vi "Build Result Array from Shots.vi"(7 "Stages":T1[](array[typedef]), 8 "Injection Event Dwell Period (ms)":dbl, 10 "Injection Event Count":u32, 11 "Shot Info Array":T5[](array[typedef]) {"Results"."Off-Stage Min Volt" format="%#.6g"; "Results"."Off-Stage Avg Volt" format="%#.6g"; "Results"."Off-Stage Max Volt" format="%#.6g"; "Results"."Total Stage Time (us)" format="%#.6g"; "Results"."Off-Stage Avg Current" format="%#.6g"; "Results"."Total Voltage Pulses" format="%#.6g"; "Results"."Off-Stage Min Current" format="%#.6g"; "Results"."Off-Stage Max Current" format="%#.6g"}) -> (1 "Result Array":dbl[](array[numeric]))   [LabVIEW 2019, in "Fuel Injector Analysis Addon Engine.lvlib"]
uses:
  Fuel Injector Analysis Addon Engine.lvlib
  RT Analysis/Controls/Shot Information Control.ctl
  Types/Stage.Measurements.ctl
  Addon Shared/Types/Stage.Parameters.ctl
  Addon Shared/Types/Stage.PullIn.Types.ctl
  Addon Shared/Types/Stage.Transition.Types.ctl
  Addon Shared/Types/Analysis.Channels.Select.ctl
  Addon Shared/Fuel Injector Analysis Addon Shared.lvlib
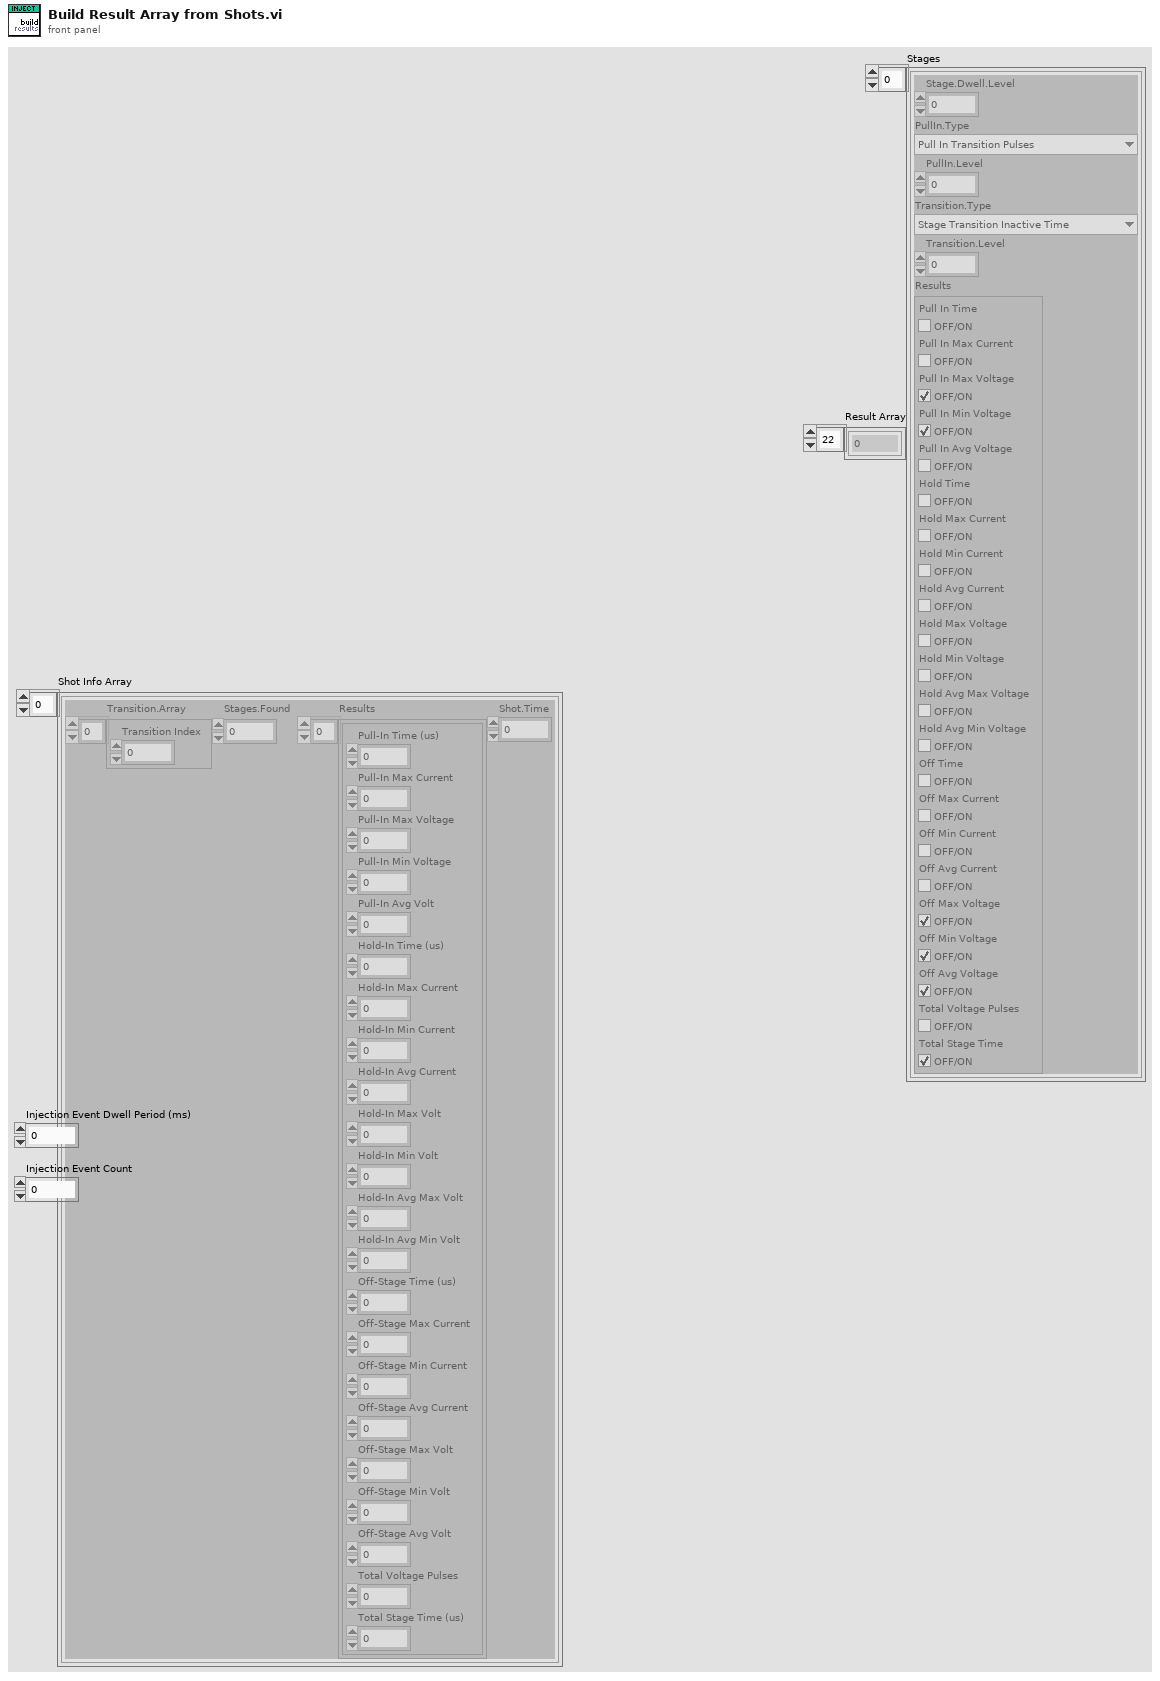
[diagram p1: front panel]
types:
  T1 = typedef "Fuel Injector Analysis Addon Shared.lvlib/Stage.Parameters.ctl" = cluster{"Stage.Dwell.Level":dbl, "PullIn.Type":T2, "PullIn.Level":dbl, "Transition.Type":T3, "Transition.Level":dbl, "Results":T4}
  T2 = typedef "Fuel Injector Analysis Addon Shared.lvlib/Stage.PullIn.Types.ctl" = enum8{"Pull In Transition Pulses", "Pull In Transition Current Drop"}
  T3 = typedef "Fuel Injector Analysis Addon Shared.lvlib/Stage.Transition.Types.ctl" = enum8{"Stage Transition Inactive Time", "Stage Transition Voltage Increase", "Stage Transition Current Decrease", "Stage Transition Active Time"}
  T4 = typedef "Fuel Injector Analysis Addon Shared.lvlib/Analysis.Channels.Select.ctl" = cluster{"Pull In Time":bool, "Pull In Max Current":bool, "Pull In Max Voltage":bool, "Pull In Min Voltage":bool, "Pull In Avg Voltage":bool, "Hold Time":bool, "Hold Max Current":bool, "Hold Min Current":bool, "Hold Avg Current":bool, "Hold Max Voltage":bool, "Hold Min Voltage":bool, "Hold Avg Max Voltage":bool, "Hold Avg Min Voltage":bool, "Off Time":bool, "Off Max Current":bool, "Off Min Current":bool, "Off Avg Current":bool, "Off Max Voltage":bool, "Off Min Voltage":bool, "Off Avg Voltage":bool, "Total Voltage Pulses":bool, "Total Stage Time":bool}
  T5 = typedef "Fuel Injector Analysis Addon Engine.lvlib/Shot Information Control.ctl" = cluster{"Transition.Array":i32[], "Stages.Found":u16, "Results":T6[], "Shot.Time":dbl}
  T6 = typedef "Fuel Injector Analysis Addon Engine.lvlib/Stage.Measurements.ctl" = cluster{"Pull-In Time (us)":dbl, "Pull-In Max Current":dbl, "Pull-In Max Voltage":dbl, "Pull-In Min Voltage":dbl, "Pull-In Avg Volt":dbl, "Hold-In Time (us)":dbl, "Hold-In Max Current":dbl, "Hold-In Min Current":dbl, "Hold-In Avg Current":dbl, "Hold-In Max Volt":dbl, "Hold-In Min Volt":dbl, "Hold-In Avg Max Volt":dbl, "Hold-In Avg Min Volt":dbl, "Off-Stage Time (us)":dbl, "Off-Stage Max Current":dbl, "Off-Stage Min Current":dbl, "Off-Stage Avg Current":dbl, "Off-Stage Max Volt":dbl, "Off-Stage Min Volt":dbl, "Off-Stage Avg Volt":dbl, "Total Voltage Pulses":dbl, "Total Stage Time (us)":dbl}
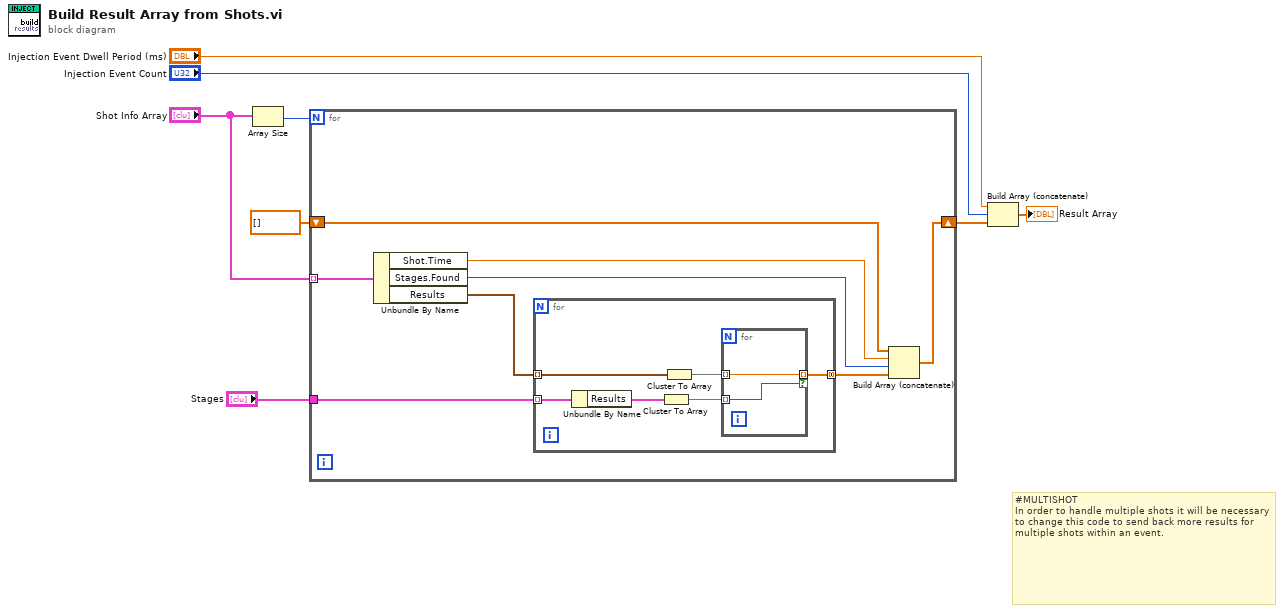
[diagram p0: block diagram]
diagram:
  # "#MULTISHOT\nIn order to handle multiple shots it will be necessary to change this code to send back more results for multiple shots within an event."
  n1 = Array Size(array="Shot Info Array") -> (size(s)=w8:i32)
  n2 = for {
    N: w8 -> [_]
    tunnel: "Shot Info Array" -> [w16] mode=indexing
    tunnel: "Stages" -> [w14]
    shift-right: [w12] -> w1
    shift-left: dbl[] [] -> [w9]
    n3 = Unbundle By Name(w16) -> ("Shot.Time"=w13:dbl, "Stages.Found"=w10:u16, "Results"=w15:T6[])
    n4 = for {
      tunnel: w15 -> [w21] mode=indexing
      tunnel: w14 -> [w22] mode=indexing
      tunnel: [w18] -> w11 mode=concatenating
      n5 = Unbundle By Name(w22) -> ("Results"=w17:T4)
      n6 = Cluster To Array(cluster=w17) -> (array=w19:bool[])
      n7 = Cluster To Array(cluster=w21) -> (array=w20:dbl[])
      n8 = for {
        tunnel: w20 -> [w24] mode=indexing
        tunnel: w19 -> [w23] mode=indexing
        tunnel: [w24] -> w18 mode=indexing if=w23
      }
    }
    n9 = Build Array (concatenate)(w9, w13, w10, w11) -> (w12:dbl[])
  }
  n10 = Build Array (concatenate)("Injection Event Dwell Period (ms)", "Injection Event Count", w1) -> (→"Result Array":dbl[])
